vi "GPS Map Graph.vi"(7 "Map config":T2={"Config path"=path "E:/Dropbox/Condivise/Condivisa con Fausto Petruzzelli/Test/GPS/Test_gps_3/mappa1.txt", "Image path"=path "E:/Dropbox/Condivise/Condivisa con Fausto Petruzzelli/Test/GPS/Test_gps_3/mappa1.png"}, 8 "Error In":errorcluster, 9 "Function":T4, 10 "Coordinates":T3, 11 "Map ref in":refnum<vi>) -> (0 "Error Out":errorcluster, 3 "Map ref out":refnum<vi>)   [LabVIEW 2015, in "My Graphs.lvlib"]
uses:
  My Graphs/My Graphs.lvlib
  My Graphs/Gps Map Graph enum.ctl
  My Graphs/Gps Map Graph coordinates.ctl
  My Graphs/Gps Map Graph config.ctl
  <vilib>/Utility/config.llb/Read Key (Double).vi
  <vilib>/Utility/config.llb/NI_LVConfig.lvlib
panel:
  in  "Coursor config":T1={"Name"="Car", "Color"=16724266, "Style"=4, "Point Style"=8, "Name Visible"=FALSE, "Allow Drag"=FALSE, "Cursor Mode"=0, "Plot"=0, "Index"=0, "Position"={"X"=765900.0, "Y"=4506130.0}, "X Scale"=0, "Y Scale"=0, "Watch Plots"=[], "Watch All Plots"=FALSE, "Plot Area"=0, "Label Offset"={"X"=0.0, "Y"=0.0}}
  out "Test map":cluster{"X":dbl, "Y":dbl}[](graph)
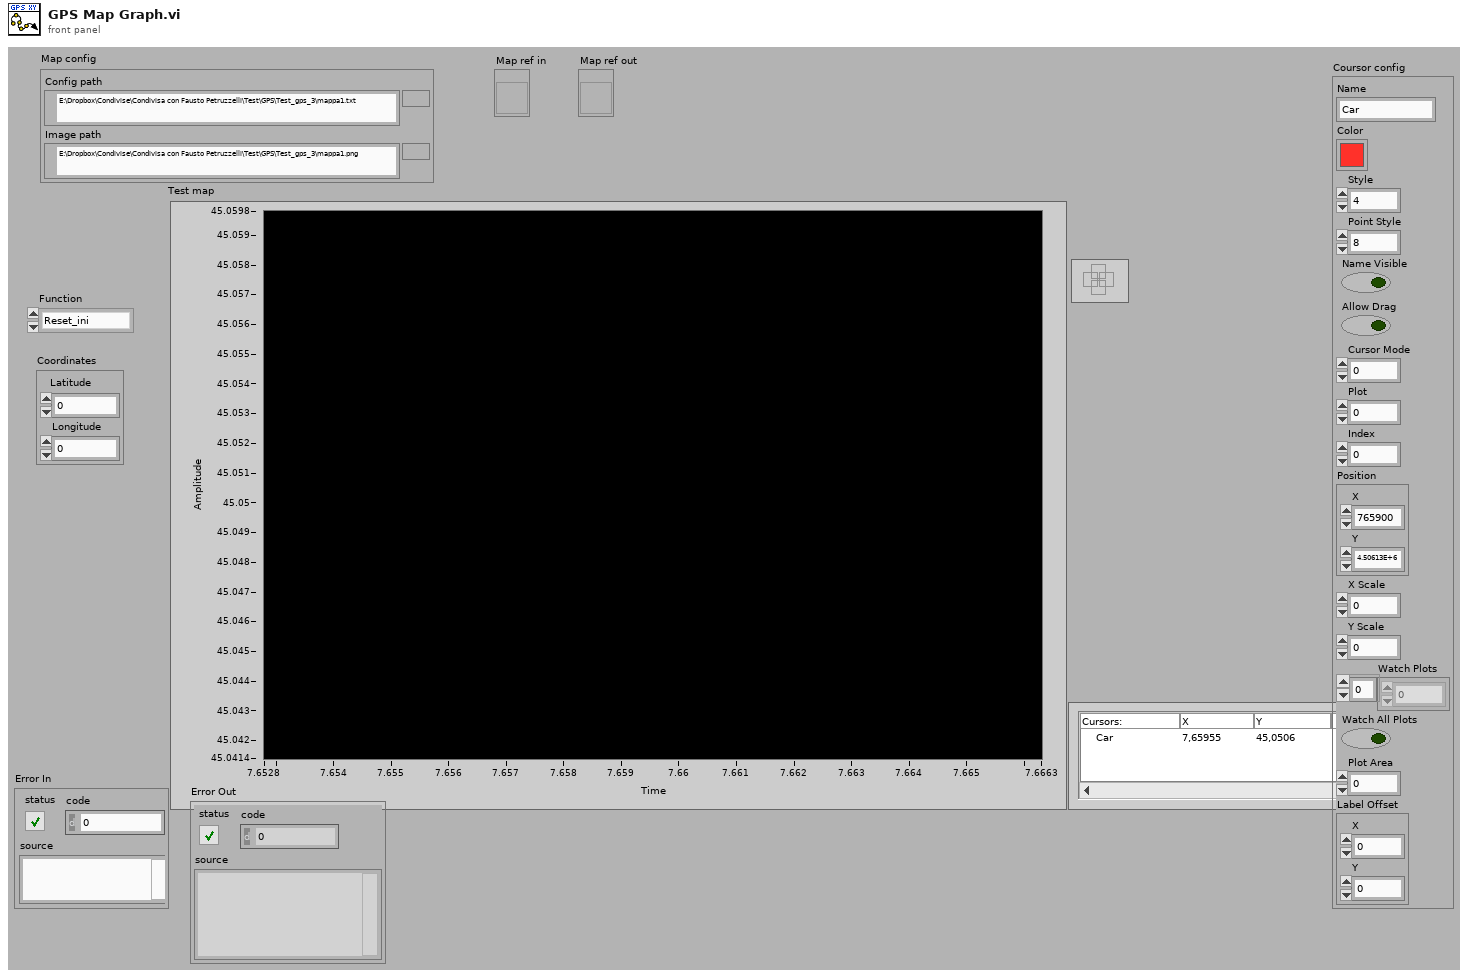
[diagram p1: front panel]
types:
  T1 = cluster{"Name":string, "Color":u32, "Style":u8, "Point Style":u8, "Name Visible":bool, "Allow Drag":bool, "Cursor Mode":u32, "Plot":i32, "Index":i32, "Position":cluster{"X":dbl, "Y":dbl}, "X Scale":u32, "Y Scale":u32, "Watch Plots":i32[], "Watch All Plots":bool, "Plot Area":i32, "Label Offset":cluster{"X":dbl, "Y":dbl}}
  T2 = typedef "Gps Map Graph config.ctl" = cluster{"Config path":path, "Image path":path}
  T3 = typedef "Gps Map Graph coordinates.ctl" = cluster{"Latitude":dbl, "Longitude":dbl}
  T4 = typedef "My Graphs.lvlib/Gps Map Graph enum.ctl" = enum16{"Reset_ini", "Reset_txt", "SetValue"}
  T5 = cluster{"Top":dbl, "Bottom":dbl, "Right":dbl, "Left":dbl}
  T6 = enum16{"open", "replace", "create", "open or create", "replace or create", "replace or create with confirmation"}
  T7 = typedef "NI_LVConfig.lvlib/Config Data RefNum.ctl" = refnum<k1>
  T8 = typedef "imagedata.ctl" = cluster{"image type":i32, "image depth":i32, "image":u8[], "mask":u8[], "colors":u32[], "Rectangle":cluster{"left":i16, "top":i16, "right":i16, "bottom":i16}}
  T9 = cluster{"Name":string, "Color":u32, "Style":u8, "Point Style":u8, "Name Visible":bool, "Allow Drag":bool, "Cursor Mode":u32, "Plot":i32, "Index":i32, "Position":cluster{"X":dbl, "Y":dbl}, "X Scale":u32, "Y Scale":u32, "Watch Plots":i32[], "Watch All Plots":bool, "Plot Area":i32, "Label Offset":cluster{"X":dbl, "Y":dbl}}[]
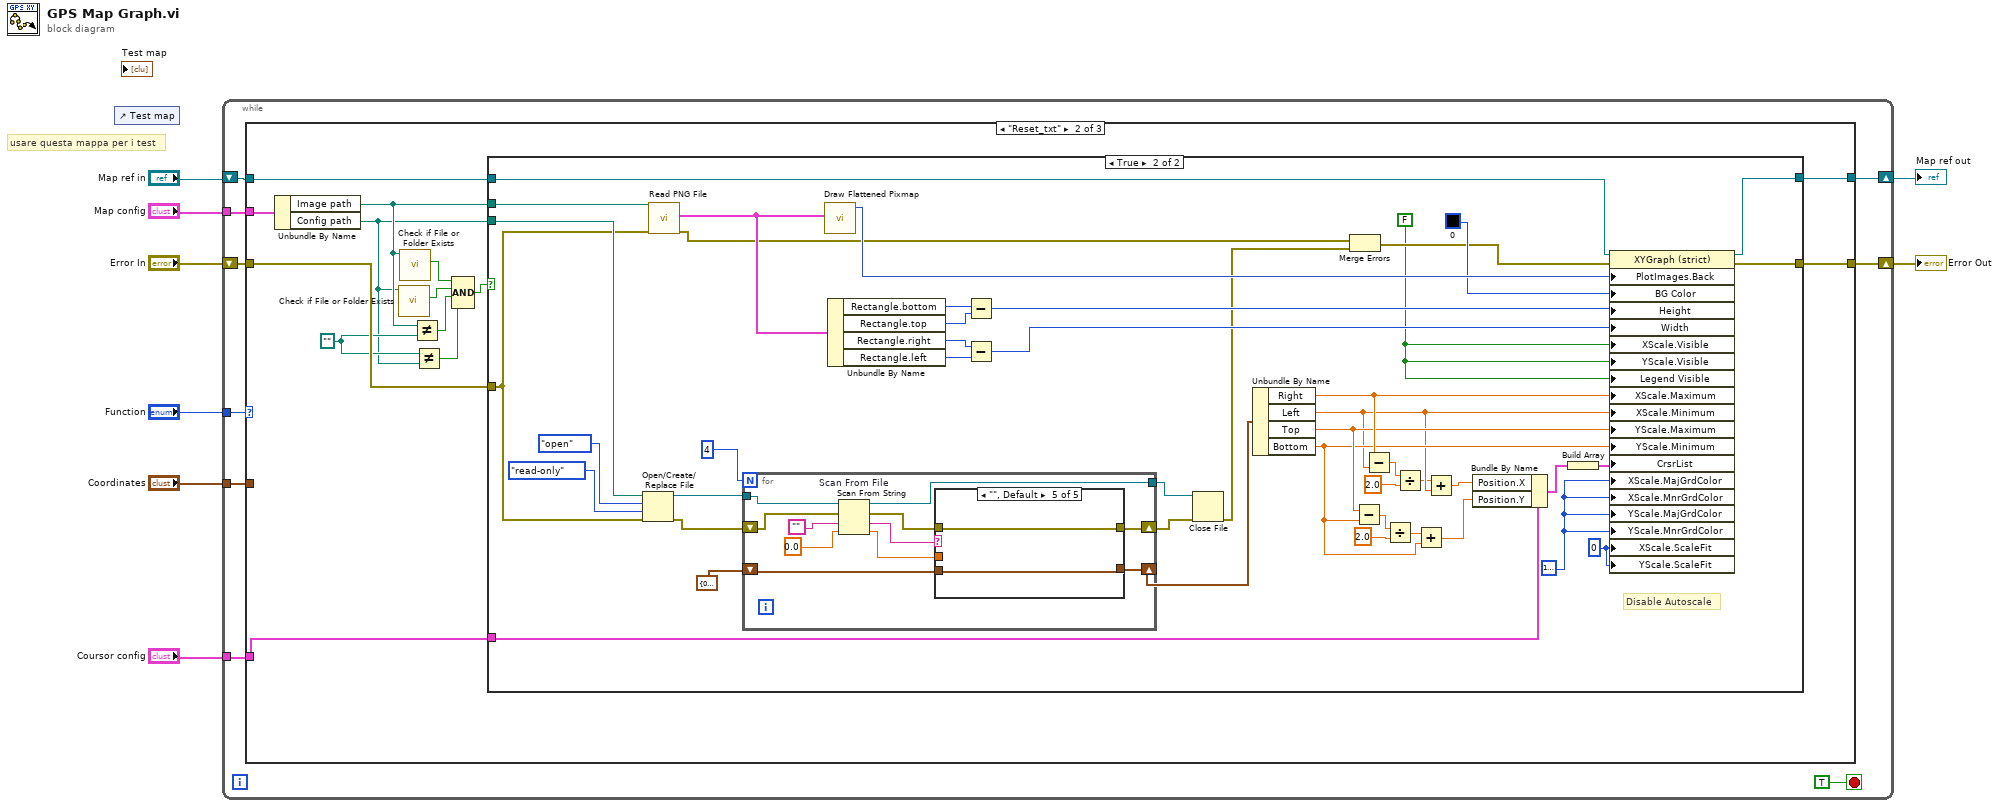
[diagram p0: block diagram]
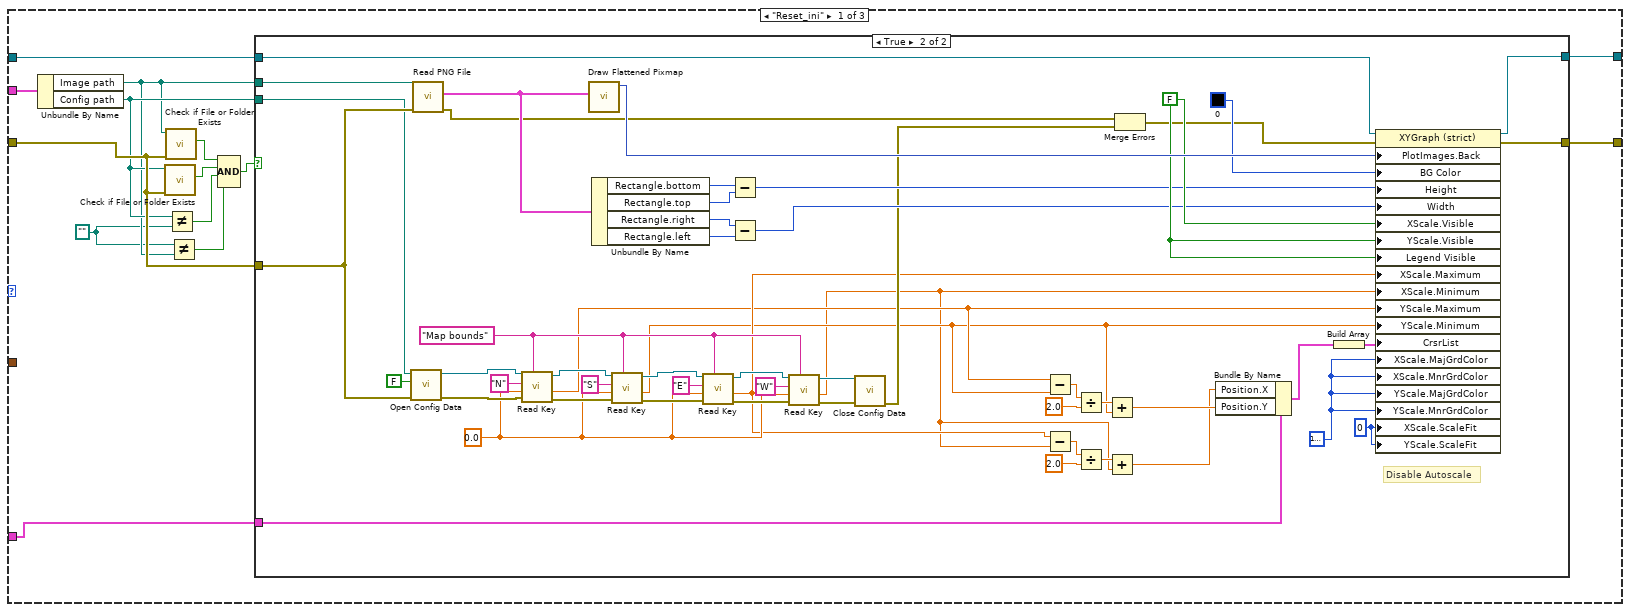
[diagram p2: hidden frame]
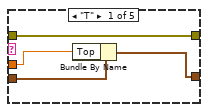
[diagram p5: hidden frame]
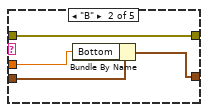
[diagram p6: hidden frame]
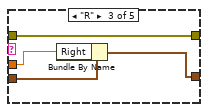
[diagram p7: hidden frame]
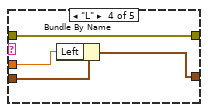
[diagram p8: hidden frame]
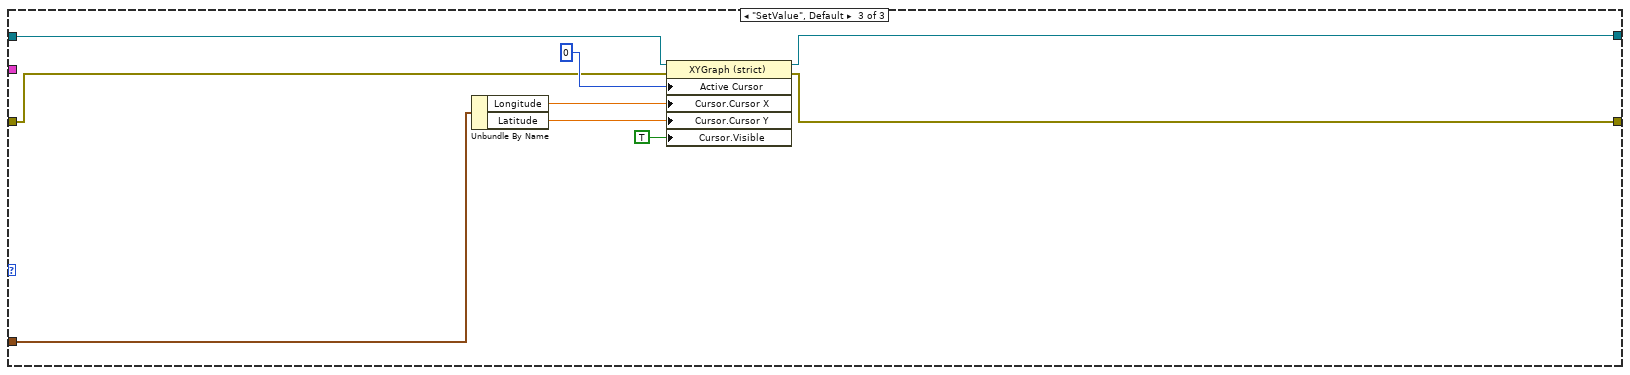
[diagram p9: hidden frame]
diagram:
  # "usare questa mappa per i test"
  n1 = control-ref of="Test map"() -> ()  [unwired: 1 out]
  n2 = while {
    tunnel: "Function" -> [w15]
    tunnel: "Coordinates" -> [w14]
    tunnel: "Map config" -> [w13]
    tunnel: "Coursor config" -> [w11]
    shift-right: [w17] -> w8
    shift-left: "Error In" -> [w16]
    shift-right: [w12] -> w3
    shift-left: "Map ref in" -> [w10]
    stop <- TRUE stop-if-true
    n3 = case shown="\"Reset_txt\"" w15 {
      tunnel: [w31 w100 w182] -> w17
      tunnel: w16 -> [w23 w99 w183]
      tunnel: w10 -> [w30 w98 w184]
      tunnel: w14 -> [_ _ w177]
      tunnel: w13 -> [w29 w97 _]
      tunnel: [w28 w96 w178] -> w12
      tunnel: w11 -> [w24 w92 _]
      frame "Reset_ini" {
        w18 = path ""
        n4 = Unbundle By Name(w29) -> ("Image path"=w19:path, "Config path"=w22:path)
        n5 = call <vilib>:"Check if File or Folder Exists.vi"("error in (no error)"=w23, "path"=w22) -> ("file or folder exists?"=w26:bool)  [unwired: 7 in, 2 out]
        n6 = call <vilib>:"Check if File or Folder Exists.vi"("error in (no error)"=w23, "path"=w19) -> ("file or folder exists?"=w25:bool)  [unwired: 7 in, 2 out]
        n7 = Not Equal?(x=w22, y=w18) -> (x != y?=w21:bool)
        n8 = Not Equal?(x=w18, y=w19) -> (x != y?=w20:bool)
        n9 = Compound Arithmetic op=AND(w25, w26, w21, w20) -> (w27:bool)
        n10 = case shown="True" w27 {
          tunnel: [w33 w74] -> w31
          tunnel: w23 -> [w33 w68]
          tunnel: w30 -> [w32 w73]
          tunnel: [w32 w71] -> w28
          tunnel: w22 -> [_ w67]
          tunnel: w19 -> [_ w70]
          tunnel: w24 -> [_ w48]
          frame False {
          }
          frame True {
            w34 = u8 0 ("X Scale.Scale Fit")
            w49 = u32 16777216
            w50 = "Map bounds" ("section")
            w55 = 0.0 ("default value")
            w84 = FALSE ("X Scale.Visible")
            # "Disable Autoscale"
            n11 = call <vilib>:"Open Config Data.vi"("error in (no error)"=w68, "create file if necessary (T)"=FALSE, "configuration file path"=w67) -> ("error out"=w56:errorcluster, "refnum"=w65:T7)  [unwired: 6 in, 1 out]
            n12 = call <vilib>:"Read PNG File.vi"("error in (no error)"=w68, "path to PNG file"=w70) -> ("error out"=w75:errorcluster, "image data"=w83:T8)  [unwired: 7 in, 1 out]
            n13 = call-poly <vilib>:"Read Key.vi"("section"=w50, "error in (no error)"=w56, "default value"=w55, "key"="N", "refnum"=w65) -> ("error out"=w57:errorcluster, "value"=w45:dbl, "refnum out"=w64:T7)  [unwired: 3 in, 1 out]
            n14 = call <vilib>:"Draw Flattened Pixmap.vi"("image data"=w83) -> ("new picture"=w86:picture)  [unwired: 8 in]
            n15 = Unbundle By Name(w83) -> ("Rectangle.bottom"=w82:i16, "Rectangle.top"=w81:i16, "Rectangle.right"=w80:i16, "Rectangle.left"=w79:i16)
            n16 = call-poly <vilib>:"Read Key.vi"("section"=w50, "error in (no error)"=w57, "default value"=w55, "key"="S", "refnum"=w64) -> ("error out"=w58:errorcluster, "value"=w38:dbl, "refnum out"=w63:T7)  [unwired: 3 in, 1 out]
            n17 = call-poly <vilib>:"Read Key.vi"("section"=w50, "error in (no error)"=w58, "default value"=w55, "key"="E", "refnum"=w63) -> ("error out"=w59:errorcluster, "value"=w46:dbl, "refnum out"=w62:T7)  [unwired: 3 in, 1 out]
            n18 = Subtract(x=w82, y=w81) -> (x-y=w78:i16)
            n19 = Subtract(x=w80, y=w79) -> (x-y=w77:i16)
            n20 = call-poly <vilib>:"Read Key.vi"("section"=w50, "error in (no error)"=w59, "default value"=w55, "key"="W", "refnum"=w62) -> ("error out"=w60:errorcluster, "value"=w35:dbl, "refnum out"=w61:T7)  [unwired: 3 in, 1 out]
            n21 = call <vilib>:"Close Config Data.vi"("error in (no error)"=w60, "refnum"=w61) -> ("error out"=w69:errorcluster)  [unwired: 8 in, 1 out]
            n22 = Subtract(x=w45, y=w38) -> (x-y=w43:dbl)
            n23 = Subtract(x=w46, y=w35) -> (x-y=w44:dbl)
            n24 = Divide(x=w43, y=2.0) -> (x/y=w40:dbl)
            n25 = Divide(x=w44, y=2.0) -> (x/y=w37:dbl)
            n26 = Add(x=w40, y=w38) -> (x+y=w39:dbl)
            n27 = Add(x=w37, y=w35) -> (x+y=w36:dbl)
            n28 = Merge Errors(w75, w69) -> (w76:errorcluster)
            n29 = Bundle By Name(cluster=w48, "Position.X"=w36, "Position.Y"=w39) -> (w47:T1)
            n30 = Build Array(w47) -> (w72:T9)
            n31 = property on="Property Node" class="XYGraph (strict)"(reference=w73, error in=w76, "PlotImages.Back"=w86, "BG Color"=u32 0, "Height"=w78, "Width"=w77, "XScale.Visible"=w84, "YScale.Visible"=w84, "Legend Visible"=w84, "XScale.Maximum"=w46, "XScale.Minimum"=w35, "YScale.Maximum"=w45, "YScale.Minimum"=w38, "CrsrList"=w72, "XScale.MajGrdColor"=w49, "XScale.MnrGrdColor"=w49, "YScale.MajGrdColor"=w49, "YScale.MnrGrdColor"=w49, "XScale.ScaleFit"=w34, "YScale.ScaleFit"=w34) -> (reference out=w71:refnum<vi>, error out=w74:errorcluster)
          }
        }
      }
      frame "Reset_txt" {
        w91 = path ""
        n32 = Unbundle By Name(w97) -> ("Image path"=w88:path, "Config path"=w87:path)
        n33 = call <vilib>:"Check if File or Folder Exists.vi"("path"=w87) -> ("file or folder exists?"=w94:bool)  [unwired: 8 in, 2 out]
        n34 = call <vilib>:"Check if File or Folder Exists.vi"("path"=w88) -> ("file or folder exists?"=w93:bool)  [unwired: 8 in, 2 out]
        n35 = Not Equal?(x=w88, y=w91) -> (x != y?=w90:bool)
        n36 = Not Equal?(x=w91, y=w87) -> (x != y?=w89:bool)
        n37 = Compound Arithmetic op=AND(w93, w94, w90, w89) -> (w95:bool)
        n38 = case shown="True" w95 {
          tunnel: [w102 w126] -> w100
          tunnel: w99 -> [w102 w115]
          tunnel: w98 -> [w101 w125]
          tunnel: [w101 w123] -> w96
          tunnel: w87 -> [_ w122]
          tunnel: w88 -> [_ w121]
          tunnel: w92 -> [_ w119]
          frame False {
          }
          frame True {
            w104 = u8 0 ("X Scale.Scale Fit")
            w120 = u32 16777216
            w103 = FALSE ("X Scale.Visible")
            # "Disable Autoscale"
            n39 = Open/Create/Replace File(file path (use dialog)=w122, error in=w115, operation (0:open)=T6."open", access (0:read/write)=enum16{"read/write", "read-only", "write-only"}."read-only") -> (refnum out=w136:refnum<file>, error out=w135:errorcluster)  [unwired: 2 in, 1 out]
            n40 = call <vilib>:"Read PNG File.vi"("error in (no error)"=w115, "path to PNG file"=w121) -> ("error out"=w127:errorcluster, "image data"=w145:T8)  [unwired: 7 in, 1 out]
            n41 = for {
              N: 4 -> [_]
              tunnel: w136 -> [w158]
              shift-right: [w151] -> w130
              shift-left: T5 {"Top"=0.0, "Bottom"=0.0, "Right"=0.0, "Left"=0.0} -> [w152]
              shift-right: [w150] -> w132
              shift-left: w135 -> [w157]
              tunnel: [w149] -> w131
              n42 = Scan From String "Scan From File"(w158, w157, default 1="", default 2=0.0) -> (w149:refnum<file>, w153:errorcluster, output 1=w155:string, output 2=w154:dbl)  [unwired: 1 in]
              n43 = case shown="\"\", Default" w155 {
                tunnel: w154 -> [w161 w164 w168 w172 _]
                tunnel: w153 -> [w159 w166 w170 w174 w176]
                tunnel: w152 -> [w162 w165 w169 w173 w175]
                tunnel: [w160 w163 w167 w171 w175] -> w151
                tunnel: [w159 w166 w170 w174 w176] -> w150
                frame "T" {
                  n44 = Bundle By Name(cluster=w162, "Top"=w161) -> (w160:T5)
                }
                frame "B" {
                  n45 = Bundle By Name(cluster=w165, "Bottom"=w164) -> (w163:T5)
                }
                frame "R" {
                  n46 = Bundle By Name(cluster=w169, "Right"=w168) -> (w167:T5)
                }
                frame "L" {
                  n47 = Bundle By Name(cluster=w173, "Left"=w172) -> (w171:T5)
                }
                frame "", Default {
                }
              }
            }
            n48 = call <vilib>:"Draw Flattened Pixmap.vi"("image data"=w145) -> ("new picture"=w147:picture)  [unwired: 8 in]
            n49 = Unbundle By Name(w145) -> ("Rectangle.bottom"=w144:i16, "Rectangle.top"=w143:i16, "Rectangle.right"=w142:i16, "Rectangle.left"=w141:i16)
            n50 = Subtract(x=w144, y=w143) -> (x-y=w140:i16)
            n51 = Subtract(x=w142, y=w141) -> (x-y=w139:i16)
            n52 = Close File(refnum=w131, error in=w132) -> (error out=w128:errorcluster)  [unwired: 1 out]
            n53 = Unbundle By Name(w130) -> ("Right"=w117:dbl, "Left"=w111:dbl, "Top"=w116:dbl, "Bottom"=w112:dbl)
            n54 = Merge Errors(w127, w128) -> (w129:errorcluster)
            n55 = Subtract(x=w116, y=w112) -> (x-y=w110:dbl)
            n56 = Subtract(x=w117, y=w111) -> (x-y=w107:dbl)
            n57 = Divide(x=w110, y=2.0) -> (x/y=w108:dbl)
            n58 = Divide(x=w107, y=2.0) -> (x/y=w106:dbl)
            n59 = Add(x=w108, y=w112) -> (x+y=w113:dbl)
            n60 = Add(x=w106, y=w111) -> (x+y=w114:dbl)
            n61 = Bundle By Name(cluster=w119, "Position.X"=w114, "Position.Y"=w113) -> (w118:T1)
            n62 = Build Array(w118) -> (w124:T9)
            n63 = property on="Property Node" class="XYGraph (strict)"(reference=w125, error in=w129, "PlotImages.Back"=w147, "BG Color"=u32 0, "Height"=w140, "Width"=w139, "XScale.Visible"=w103, "YScale.Visible"=w103, "Legend Visible"=w103, "XScale.Maximum"=w117, "XScale.Minimum"=w111, "YScale.Maximum"=w116, "YScale.Minimum"=w112, "CrsrList"=w124, "XScale.MajGrdColor"=w120, "XScale.MnrGrdColor"=w120, "YScale.MajGrdColor"=w120, "YScale.MnrGrdColor"=w120, "XScale.ScaleFit"=w104, "YScale.ScaleFit"=w104) -> (reference out=w123:refnum<vi>, error out=w126:errorcluster)
          }
        }
      }
      frame "SetValue", Default {
        n64 = Unbundle By Name(w177) -> ("Longitude"=w181:dbl, "Latitude"=w180:dbl)
        n65 = property class="XYGraph (strict)"(reference=w184, error in=w183, "Active Cursor"=u32 0, "Cursor.Cursor X"=w181, "Cursor.Cursor Y"=w180, "Cursor.Visible"=TRUE) -> (reference out=w178:refnum<vi>, error out=w182:errorcluster)
      }
    }
  }
  "Error Out" <- w8
  "Map ref out" <- w3
